vi "Fit Line.vi"(8 "error in (no error)":errorcluster, 11 "Points":refnum<class "Vec3d.lvclass">[](array[class])) -> (0 "error out":errorcluster, 1 "residue":dbl, 2 "intercept":dbl, 3 "slope":dbl)   [LabVIEW 2023]
uses:
  Vec3d Class/Vec3d.lvclass
  <vilib>/Analysis/6fits.llb/Curve Fitting Criteria.ctl
  <vilib>/Analysis/NI_AALPro.lvlib
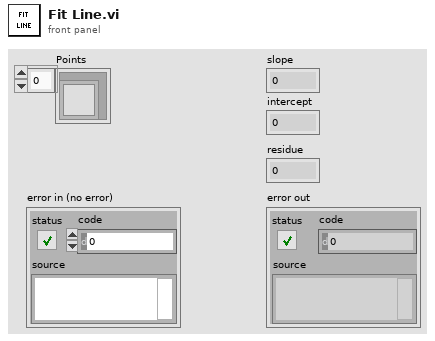
[diagram p1: front panel]
types:
  T1 = typedef "NI_AALPro.lvlib/Curve Fitting Criteria.ctl" = u16
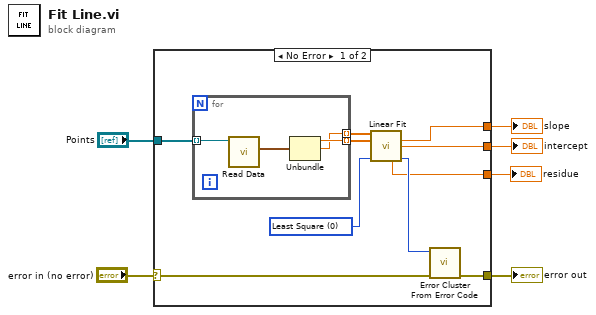
[diagram p0: block diagram]
diagram:
  n1 = case shown="No Error" "error in (no error)" {
    selector: "error in (no error)" -> [w8 w21]
    tunnel: "Points" -> [w16 _]
    tunnel: [w13 _] -> w5
    tunnel: [w12 _] -> w4
    tunnel: [w9 w21] -> w2
    tunnel: [w7 _] -> w1
    frame No Error {
      w11 = T1 0 items=["Least Square", "Least Absolute Residual", "Bisquare"] ("method")
      n2 = for {
        tunnel: w16 -> [w20] mode=indexing
        tunnel: [w18] -> w15 mode=indexing
        tunnel: [w17] -> w14 mode=indexing
        n3 = call-dynamic "Read Data.vi"("Vec3d Class in"=w20) -> ("Data"=w19:cluster{"X":dbl, "Y":dbl, "Z":dbl})  [unwired: 8 in, 2 out]
        n4 = Unbundle(w19) -> ("X"=w18:dbl, "Y"=w17:dbl)  [unwired: 1 out]
      }
      n5 = call <vilib>:"Linear Fit.vi"("Y"=w14, "X"=w15, "method"=w11) -> ("slope"=w13:dbl, "intercept"=w12:dbl, "residue"=w7:dbl, "error"=w10:i32)  [unwired: 8 in, 1 out]
      n6 = call <vilib>:"Error Cluster From Error Code.vi"("error in (no error)"=w8, "error code (0)"=w10) -> ("error out"=w9:errorcluster)  [unwired: 7 in]
    }
    frame Error {
    }
  }
  "slope" <- w5
  "intercept" <- w4
  "error out" <- w2
  "residue" <- w1
